vi "Check SPI Pins.vi"(8 "error in (no error)":errorcluster, 9 "SPI Pins":T2={"TX GPIO"=-1, "RX GPIO"=-1, "SCK GPIO"=6}, 10 "SPI #":T1=-1, 11 "Session in":refnum<class "Session.lvclass">) -> (0 "error out":errorcluster, 3 "Session out":refnum<class "Session.lvclass">)   [LabVIEW 2020, in "CTI.lvlib" / "Session.lvclass"]
uses:
  Session.lvclass
  SPI Pins.ctl
  GPIO Number.ctl
  SPI Number.ctl
  Session.lvclass/Session.ctl
  CTI.lvlib
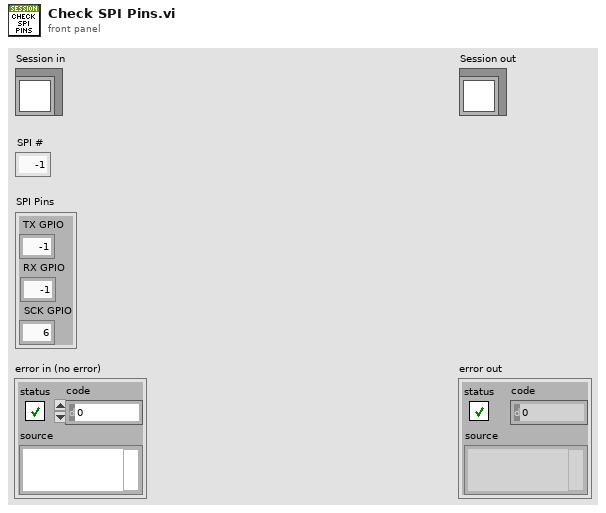
[diagram p1: front panel]
types:
  T1 = typedef "CTI.lvlib/SPI Number.ctl" = i8
  T2 = typedef "CTI.lvlib/SPI Pins.ctl" = cluster{"TX GPIO":T3, "RX GPIO":T3, "SCK GPIO":T3}
  T3 = typedef "CTI.lvlib/GPIO Number.ctl" = i8
  T4 = typedef "CTI.lvlib/Available SPI.ctl" = cluster{"SPI #":T1, "TX GPIOs":T3[], "RX GPIOs":T3[], "SCK GPIOs":T3[]}
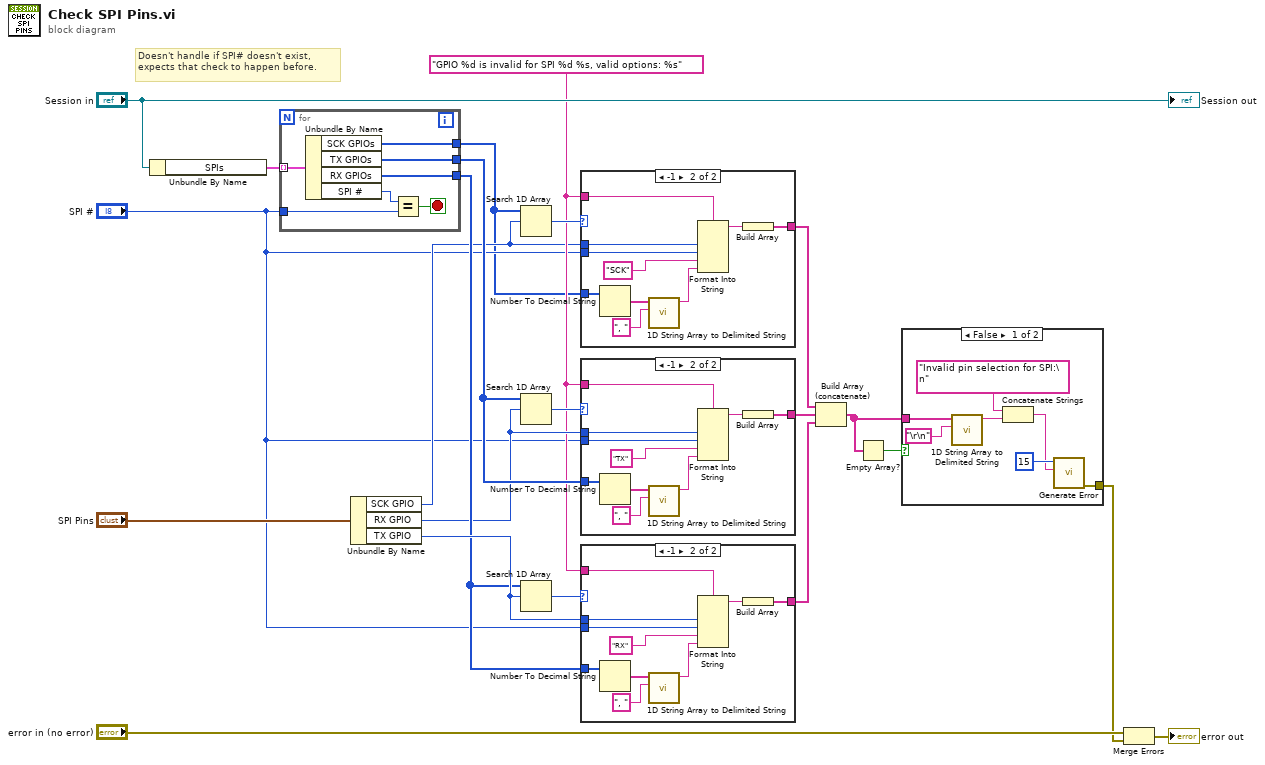
[diagram p0: block diagram]
diagram:
  w4 = "GPIO %d is invalid for SPI %d %s, valid options: %s"
  # "Doesn't handle if SPI# doesn't exist, expects that check to happen before."
  n1 = Unbundle By Name("Session in") -> ("SPIs"=w19:T4[])
  n2 = for {
    tunnel: w19 -> [w29] mode=indexing
    tunnel: "SPI #" -> [w28]
    tunnel: [w26] -> w14
    tunnel: [w25] -> w16
    tunnel: [w23] -> w1
    stop <- w24 stop-if-true
    n3 = Unbundle By Name(w29) -> ("SCK GPIOs"=w23:T3[], "TX GPIOs"=w26:T3[], "RX GPIOs"=w25:T3[], "SPI #"=w27:T1)
    n4 = Equal?(x=w27, y=w28) -> (x = y?=w24:bool)
  }
  n5 = Unbundle By Name("SPI Pins") -> ("SCK GPIO"=w3:T3, "RX GPIO"=w13:T3, "TX GPIO"=w17:T3)
  n6 = Search 1D Array(1D array=w1, element=w3) -> (index of element=w6:i32)  [unwired: 1 in]
  n7 = Search 1D Array(1D array=w14, element=w13) -> (index of element=w15:i32)  [unwired: 1 in]
  n8 = Search 1D Array(1D array=w16, element=w17) -> (index of element=w18:i32)  [unwired: 1 in]
  n9 = case shown="-1" w6 {
    tunnel: w4 -> [_ w39]
    tunnel: "SPI #" -> [_ w37]
    tunnel: w3 -> [_ w38]
    tunnel: w1 -> [_ w35]
    tunnel: [_ w30] -> w5
    frame Default {
    }
    frame -1 {
      n10 = Number To Decimal String(number=w35) -> (decimal integer string=w34:string[])  [unwired: 1 in]
      n11 = call <vilib>:"1D String Array to Delimited String.vi"("delimiter"=", ", "string array"=w34) -> ("delimited string"=w32:string)  [unwired: 9 in]
      n12 = Format Into String(format string=w39, w38, w37, "SCK" ("input 3"), w32) -> (resulting string=w31:string)  [unwired: 2 in, 1 out]
      n13 = Build Array(w31) -> (w30:string[])
    }
  }
  n14 = case shown="-1" w15 {
    tunnel: w4 -> [_ w49]
    tunnel: "SPI #" -> [_ w47]
    tunnel: w13 -> [_ w48]
    tunnel: w14 -> [_ w45]
    tunnel: [_ w40] -> w12
    frame Default {
    }
    frame -1 {
      n15 = Number To Decimal String(number=w45) -> (decimal integer string=w44:string[])  [unwired: 1 in]
      n16 = call <vilib>:"1D String Array to Delimited String.vi"("delimiter"=", ", "string array"=w44) -> ("delimited string"=w42:string)  [unwired: 9 in]
      n17 = Format Into String(format string=w49, w48, w47, "TX" ("input 3"), w42) -> (resulting string=w41:string)  [unwired: 2 in, 1 out]
      n18 = Build Array(w41) -> (w40:string[])
    }
  }
  n19 = case shown="-1" w18 {
    tunnel: w4 -> [_ w59]
    tunnel: "SPI #" -> [_ w57]
    tunnel: w17 -> [_ w58]
    tunnel: w16 -> [_ w55]
    tunnel: [_ w50] -> w11
    frame Default {
    }
    frame -1 {
      n20 = Number To Decimal String(number=w55) -> (decimal integer string=w54:string[])  [unwired: 1 in]
      n21 = call <vilib>:"1D String Array to Delimited String.vi"("delimiter"=", ", "string array"=w54) -> ("delimited string"=w52:string)  [unwired: 9 in]
      n22 = Format Into String(format string=w59, w58, w57, "RX" ("input 3"), w52) -> (resulting string=w51:string)  [unwired: 2 in, 1 out]
      n23 = Build Array(w51) -> (w50:string[])
    }
  }
  n24 = Build Array (concatenate)(w5, w12, w11) -> (w9:string[])
  n25 = Empty Array?(array=w9) -> (empty?=w10:bool)
  n26 = case shown="False" w10 {
    tunnel: w9 -> [w66 _]
    tunnel: [w63 _] -> w7
    frame False {
      n27 = call <vilib>:"1D String Array to Delimited String.vi"("delimiter"="\r\n", "string array"=w66) -> ("delimited string"=w61:string)  [unwired: 9 in]
      n28 = Concatenate Strings("Invalid pin selection for SPI:\n" ("format string"), w61) -> (w60:string)
      n29 = call "Generate Error.vi"("error message"=w60, "error code"=15) -> ("error out"=w63:errorcluster)  [unwired: 9 in]
    }
    frame True {
    }
  }
  n30 = Merge Errors("error in (no error)", w7) -> (→"error out":errorcluster)
  "Session out" <- "Session in"
